vi "改进数值比较.vi"() -> ()   [LabVIEW 2022 SP3]
doc: "本VI是为《我和LabVIEW》一书编写的示例。\n关于本书的介绍请参考网页：\nhttp://ruanqizhen.spaces.live.com/blog/cns!5852D4F797C53FB6!4310.entry"
panel:
  in  "b":i32
  in  "a":i32
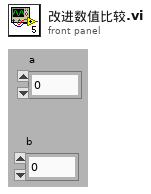
[diagram p1: front panel]
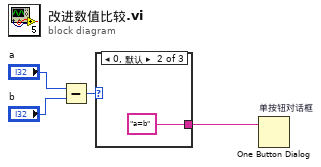
[diagram p0: block diagram]
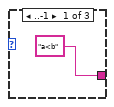
[diagram p2: hidden frame]
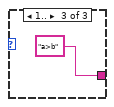
[diagram p3: hidden frame]
diagram:
  n1 = Subtract(x="a", y="b") -> (x-y=w2:i32)
  n2 = case shown="0, 默认" w2 {
    tunnel: ["a<b" "a=b" "a>b"] -> w1
    frame ..-1 {
    }
    frame 0, Default {
    }
    frame 1.. {
    }
  }
  n3 = One Button Dialog "单按钮对话框"(message=w1) -> ()  [unwired: 2 out]
